vi "Change Color.vi"(6 "Back Ground Color":u32(colorbox)=16748288, 9 "Current Color":u32(colorbox)=16748288, 11 "Color Strength (%)":dbl(slide) scale=0.0..100.0) -> (3 "output array":cluster{"Color":u32, "Color":u32}[](array[cluster]))   [LabVIEW 2014]
panel:
  out "Color":u32(colorbox)
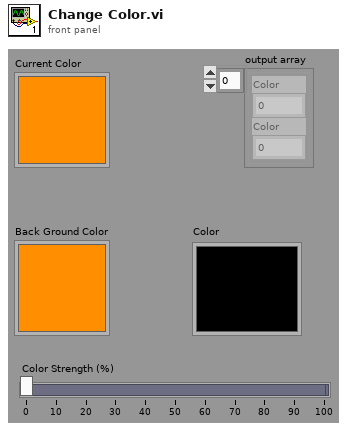
[diagram p1: front panel]
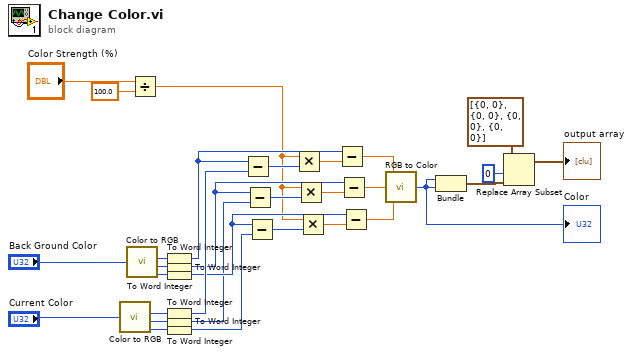
[diagram p0: block diagram]
diagram:
  n1 = call <vilib>:"Color to RGB.vi"("Color"="Current Color") -> ("R"=w19:u8, "G"=w13:u8, "B"=w12:u8)  [unwired: 1 out]
  n2 = call <vilib>:"Color to RGB.vi"("Color"="Back Ground Color") -> ("R"=w17:u8, "G"=w15:u8, "B"=w14:u8)  [unwired: 1 out]
  n3 = Divide(x="Color Strength (%)", y=100.0) -> (x/y=w3:dbl)
  n4 = To Word Integer(number=w17) -> (16bit integer=w16:i16)
  n5 = To Word Integer(number=w15) -> (16bit integer=w7:i16)
  n6 = To Word Integer(number=w14) -> (16bit integer=w6:i16)
  n7 = To Word Integer(number=w19) -> (16bit integer=w18:i16)
  n8 = To Word Integer(number=w13) -> (16bit integer=w5:i16)
  n9 = To Word Integer(number=w12) -> (16bit integer=w4:i16)
  n10 = Subtract(x=w16, y=w18) -> (x-y=w22:i16)
  n11 = Subtract(x=w7, y=w5) -> (x-y=w11:i16)
  n12 = Subtract(x=w6, y=w4) -> (x-y=w10:i16)
  n13 = Multiply(x=w3, y=w22) -> (x*y=w21:dbl)
  n14 = Multiply(x=w3, y=w11) -> (x*y=w8:dbl)
  n15 = Multiply(x=w3, y=w10) -> (x*y=w9:dbl)
  n16 = Subtract(x=w16, y=w21) -> (x-y=w20:dbl)
  n17 = Subtract(x=w7, y=w8) -> (x-y=w2:dbl)
  n18 = Subtract(x=w6, y=w9) -> (x-y=w1:dbl)
  n19 = call <vilib>:"RGB to Color.vi"("B"=w1, "G"=w2, "R"=w20) -> ("Color"=w30:u32)
  "Color" <- w30
  n20 = Bundle("Color"=w30, "Color"=w30) -> (w28:cluster{"Color":u32, "Color":u32})  [unwired: 1 out]
  n21 = Replace Array Subset(array=cluster{"Color":u32, "Color":u32}[] [{"Color"=0, "Color"=0}, {"Color"=0, "Color"=0}, {"Color"=0, "Color"=0}, {"Color"=0, "Color"=0}], new element=w28, index=0) -> (→"output array":cluster{"Color":u32, "Color":u32}[])
